vi "First Step.vi"(8 "error in (no error)":errorcluster, 11 "Translation Stage Coarse.lvclass in":refnum<class "Translation Stage Coarse.lvclass">) -> (0 "error out":errorcluster, 2 "Current Position":dbl, 3 "Translation Stage Coarse.lvclass out":refnum<class "Translation Stage Coarse.lvclass">)   [LabVIEW 2017, in "Translation Stage Coarse.lvclass"]
doc: "(Dynamic) Reset the instrument and prepare to scan. Go to step #0 - the first step. If desired, the scanner may do this in a different way than usual (i.e. by preparing to move a long distance, or reset to home position.)"
uses:
  Translation Stage Coarse.lvclass
  Global/GPIB Numbers.vi
  Scanner/Scanner.lvclass
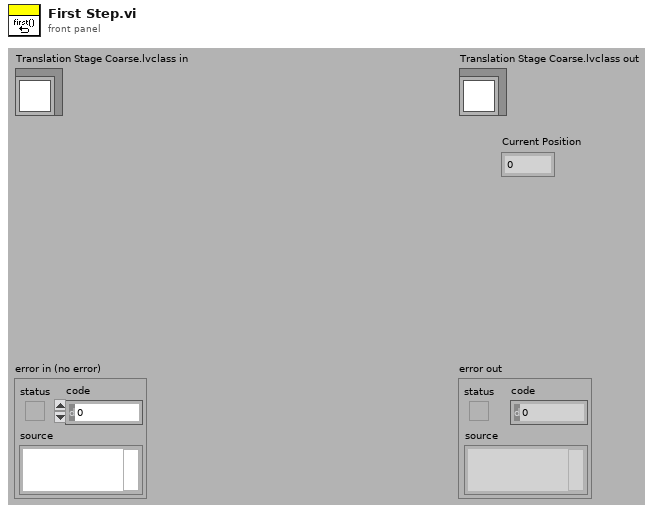
[diagram p1: front panel]
types:
  T1 = typedef "GPIB Type Def.ctl" = cluster{"Name":string, "bus":dbl, "GPIB":dbl, "GPIB as string":string, "byte":i32, "VISA Resource Name":refnum<visa-resource-name>}
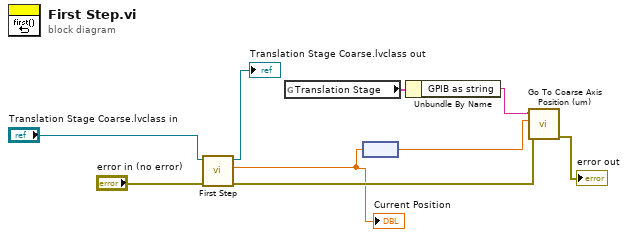
[diagram p0: block diagram]
diagram:
  n1 = call-parent "First Step.vi"("error in (no error)"="error in (no error)", "Scanner.lvclass in"="Translation Stage Coarse.lvclass in") -> ("error out"=w3:errorcluster, "Current Position"=w1:dbl, "Scanner.lvclass out"=→"Translation Stage Coarse.lvclass out":refnum<class "Translation Stage Coarse.lvclass">)  [unwired: 7 in]
  "Current Position" <- w1
  n2 = global read "GPIB Numbers.vi" "Translation Stage"() -> (w7:T1)
  n3 = node(w1) -> (w2:dbl[unit])
  n4 = Unbundle By Name(w7) -> ("GPIB as string"=w5:string)
  n5 = call "Go To Coarse Axis Position (um).vi"("error in (no error)"=w3, "Coarse Axis Position (um)"=w2, "GPIB # (in): def. 6"=w5) -> ("error out"=→"error out":errorcluster)  [unwired: 7 in, 1 out]
